vi "Player Hand History Analyzer.vi"() -> ()   [LabVIEW 2020]
panel:
  out "Card Map":T1(array[cluster]) {"Average Profit/Loss (BBs)" format="%#_3g"}
  out "Overall Profit/Loss (BBs)":dbl
  out "Total Hands":i32
  out "Shown Hands":string[](array[string])
  in  "Player":string
  # "SUITED"
  # "OFFSUIT"
  # "A"
  # "K"
  # "Q"
  # "J"
  # "T"
  # "9"
  # "8"
  # "7"
  # "6"
  # "5"
  # "4"
  # "3"
  # "2"
  # "2"
  # "3"
  # "4"
  # "5"
  # "6"
  # "7"
  # "8"
  # "9"
  # "T"
  # "J"
  # "Q"
  # "K"
  # "A"
  # "A"
  # "K"
  # "Q"
  # "J"
  # "T"
  # "9"
  # "8"
  # "7"
  # "6"
  # "5"
  # "4"
  # "3"
  # "2"
  # "2"
  # "3"
  # "4"
  # "5"
  # "6"
  # "7"
  # "8"
  # "9"
  # "T"
  # "J"
  # "Q"
  # "K"
  # "A"
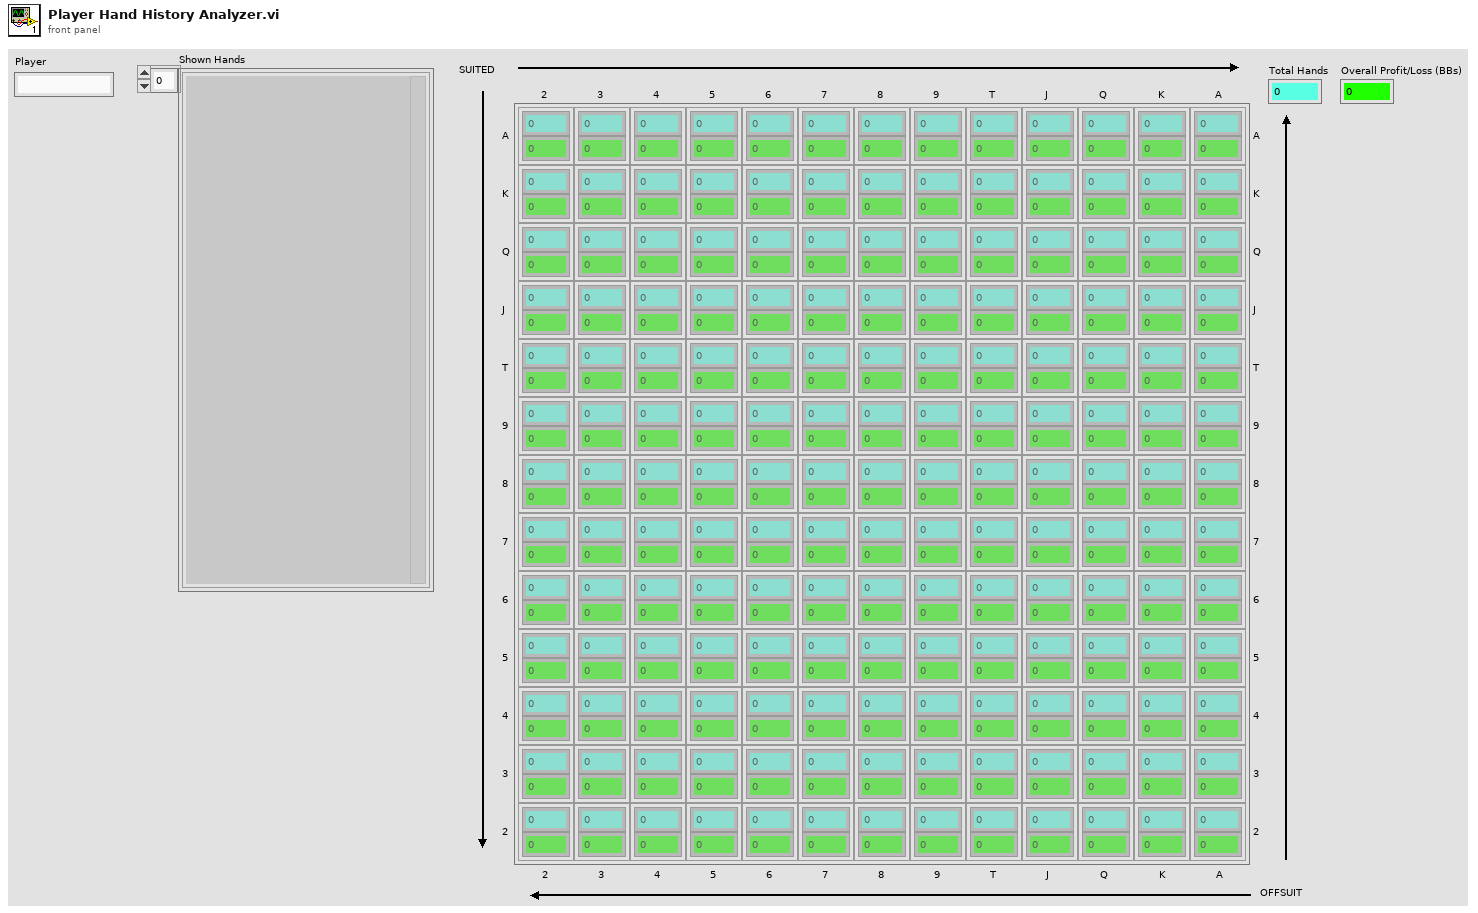
[diagram p1: front panel]
types:
  T1 = cluster{"Hand Count":u16, "Average Profit/Loss (BBs)":dbl}[][]
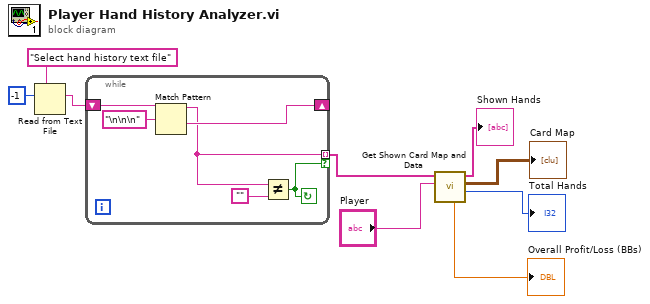
[diagram p0: block diagram]
diagram:
  n1 = Read from Text File(prompt (Open existing file)="Select hand history text file", count=-1) -> (text=w7:string)  [unwired: 2 in, 3 out]
  n2 = while {
    shift-right: [w14] -> _
    shift-left: w7 -> [w15]
    tunnel: [w12] -> w6 mode=indexing if=w10
    stop <- w10 continue-if-true
    n3 = Match Pattern(string=w15, regular expression="\n\n\n") -> (before substring=w12:string, after substring=w14:string)  [unwired: 1 in, 2 out]
    n4 = Not Equal?(x=w12, y="") -> (x != y?=w10:bool)
  }
  n5 = call "Get Shown Card Map and Data.vi"("Player"="Player", "Hand Array"=w6) -> ("Total Hands"=→"Total Hands":i32, "Card Map"=→"Card Map":T1, "Shown Hands"=→"Shown Hands":string[], "Overall Profit Loss (BBs)"=→"Overall Profit/Loss (BBs)":dbl)  [unwired: 6 in]
